vi "tc_array.vi"(0 "TC Label":string, 1 "output array 2":T1(array[cluster]), 5 "Temperature":dbl format="%#_13g", 7 "Graph ON/OFF":u32(colorbox)=4250624, 9 "Plot Color":u32(colorbox)=16860, 11 "Alarm String":string, 12 "index (row)":i32, 13 "AlarmColor":u32(colorbox)) -> (4 "output array":T1(array[cluster]))   [LabVIEW 2016]
panel:
  in  "index (col)":i32
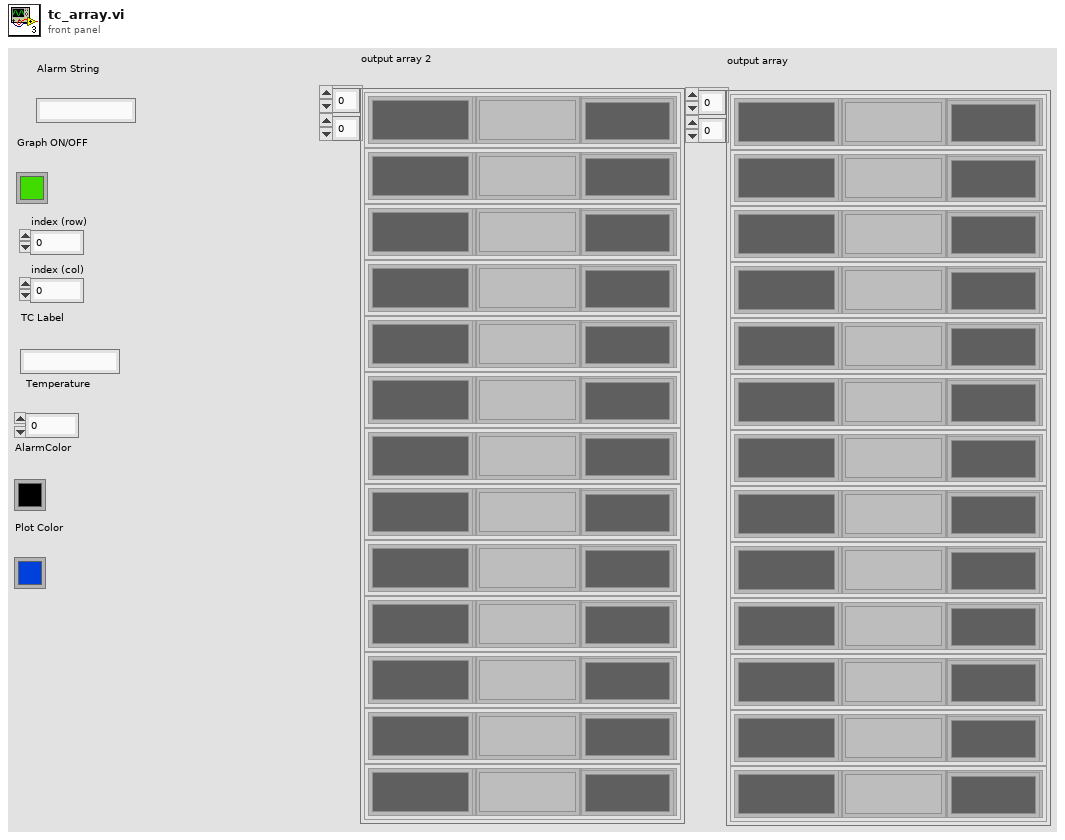
[diagram p1: front panel]
types:
  T1 = cluster{"TC Label":string, "Alarm Status":string, "Alarm Color":u32, "Temperature":string, "PlotColor":u32, "Graph On/Off":u32}[][]
  T2 = cluster{"TC Label":string, "Alarm Status":string, "Alarm Color":u32, "Temperature":string, "PlotColor":u32, "Graph On/Off":u32}
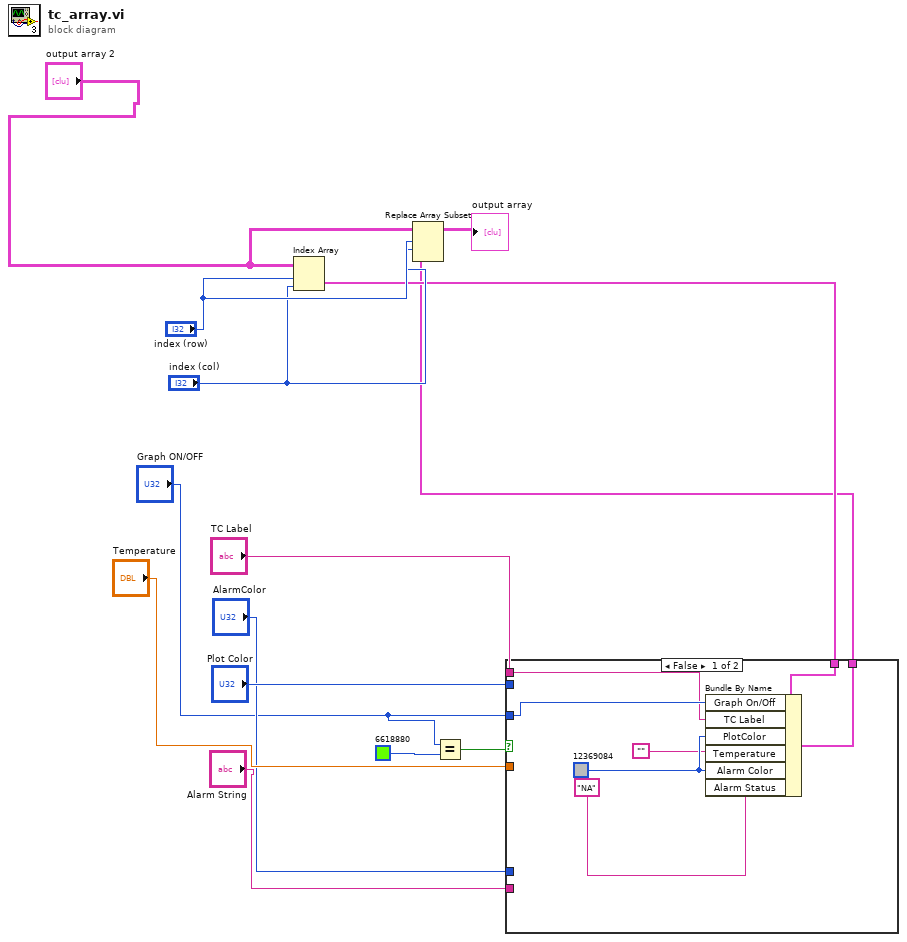
[diagram p0: block diagram]
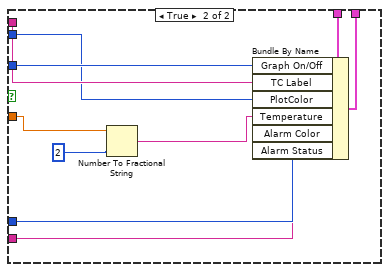
[diagram p2: hidden frame]
diagram:
  n1 = Index Array(array="output array 2", index (row)="index (row)", index (col)="index (col)") -> (element=w12:T2)
  n2 = Equal?(x="Graph ON/OFF", y=u32 6618880) -> (x = y?=w3:bool)
  n3 = case shown="False" w3 {
    tunnel: w12 -> [w21 w31]
    tunnel: "Graph ON/OFF" -> [w19 w30]
    tunnel: "TC Label" -> [w16 w29]
    tunnel: "Plot Color" -> [_ w28]
    tunnel: "Temperature" -> [_ w24]
    tunnel: "AlarmColor" -> [_ w27]
    tunnel: "Alarm String" -> [_ w26]
    tunnel: [w20 w25] -> w6
    frame False {
      w17 = u32 12369084 ("Alarm Color")
      n4 = Bundle By Name(cluster=w21, "Graph On/Off"=w19, "TC Label"=w16, "PlotColor"=w17, "Temperature"="", "Alarm Color"=w17, "Alarm Status"="NA") -> (w20:T2)
    }
    frame True {
      n5 = Number To Fractional String(number=w24, precision (6)=i16 2 ("width (-)")) -> (F-format string=w23:string)  [unwired: 2 in]
      n6 = Bundle By Name(cluster=w31, "Graph On/Off"=w30, "TC Label"=w29, "PlotColor"=w28, "Temperature"=w23, "Alarm Color"=w27, "Alarm Status"=w26) -> (w25:T2)
    }
  }
  n7 = Replace Array Subset(array="output array 2", new element=w6, index (row)="index (row)", index (col)="index (col)") -> (→"output array":T1)
